vi "Create PID Controller.vi"() -> ()   [LabVIEW 2013, in "Control SysDef API.lvlib"]
uses:
  Control SysDef API.lvlib
  NationalInstruments.VeriStand.SystemDefinitionAPI
  System Explorer/Control Addon System Explorer.lvlib
  Shared/Control Addon Shared.lvlib
  Shared/Types/Action.ctl
  Shared/Constants.vi
panel:
  out "error out":errorcluster
  in  "error in (no error)":errorcluster
  in  "Custom Device Ref":refnum<k24>
  out "Custom Device Ref":refnum<k24>
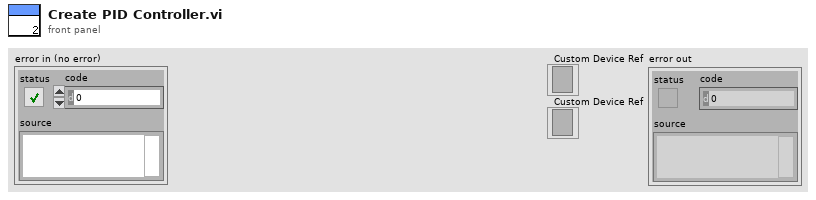
[diagram p1: front panel]
types:
  T1 = typedef "Control Addon Shared.lvlib/Action.ctl" = enum16{"Get", "Set"}
  T2 = typedef "Custom Device API.lvlib/Custom Device Item Ref.ctl" = u64
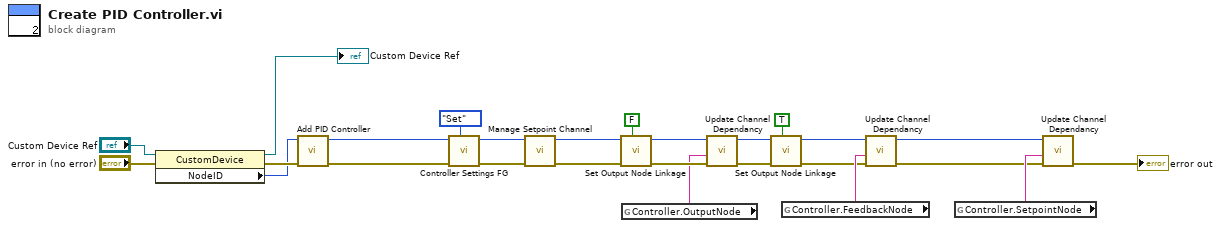
[diagram p0: block diagram]
diagram:
  n1 = property class="CustomDevice"(reference="Custom Device Ref", error in="error in (no error)") -> (reference out=→"Custom Device Ref":refnum<k24>, error out=w27:errorcluster, "NodeID"=w12:u64)
  n2 = call "Add PID Controller.vi"("error in (no error)"=w27, "Node Ptr"=w12) -> ("error out"=w13:errorcluster, "Controller Ref Out"=w1:T2)  [unwired: 7 in, 1 out]
  n3 = call "Controller Settings FG.vi"("Action"=Action."Set", "error in (no error)"=w13, "Node Ptr"=w1) -> ("error out"=w10:errorcluster, "Item Ref out"=w11:T2)  [unwired: 6 in, 1 out]
  n4 = call "Manage Setpoint Channel.vi"("error in (no error)"=w10, "Node Ptr"=w11) -> ("error out"=w9:errorcluster, "Node Ptr out"=w8:T2)  [unwired: 8 in]
  n5 = call "Set Output Node Linkage.vi"("Add?"=FALSE, "error in"=w9, "Section Ref in"=w8) -> ("error out"=w23:errorcluster, "Item Ref out"=w24:T2)  [unwired: 7 in]
  n6 = global read "Constants.vi" "Controller.OutputNode"() -> (w18:string)
  n7 = call "Update Channel Dependancy.vi"("error in (no error)"=w23, "NodeName"=w18, "Item Ref in"=w24) -> ("error out"=w19:errorcluster, "Item Ref out"=w20:T2, "Data"=w17:variant)  [unwired: 6 in]
  n8 = call "Set Output Node Linkage.vi"("Add?"=TRUE, "error in"=w19, "Section Ref in"=w20) -> ("error out"=w6:errorcluster, "Item Ref out"=w5:T2)  [unwired: 7 in]
  n9 = global read "Constants.vi" "Controller.FeedbackNode"() -> (w14:string)
  n10 = call "Update Channel Dependancy.vi"("error in (no error)"=w6, "NodeName"=w14, "Item Ref in"=w5) -> ("error out"=w4:errorcluster, "Item Ref out"=w3:T2, "Data"=w7:variant)  [unwired: 6 in]
  n11 = global read "Constants.vi" "Controller.SetpointNode"() -> (w16:string)
  n12 = call "Update Channel Dependancy.vi"("error in (no error)"=w4, "NodeName"=w16, "Item Ref in"=w3) -> ("error out"=→"error out":errorcluster, "Data"=w15:variant)  [unwired: 6 in, 1 out]
